vi "GetCmapArrays.vi"() -> (0 "Parula Array":u32[](array[numeric])=[4073128, 4073388, 4139183, 4139442, 4205236, 4205495, 4271290, 4271549, 4337343, 4337602, 4403397, 4403656, 4403914, 4469709, 4469968, 4535762, 4536277, 4536535, 4602329, 4602588, 4602846, 4603360, 4669153, 4669411, 4669925, 4670182, 4670696, 4670953, 4671211, 4737260, 4737517, 4738030, 4738288, 4738801, 4739058, 4739315, 4739828, 4740085, 4740342, 4675319, 4675575, 4676088, 4676345, 4676602, 4677114, 4611835, 4612347, 4612604, 4547324, 4547837, 4482557, 4417533, 4417790, 4352766, 4287486, 4222462, 4157183, 4092159, 3961343, 3896319, 3765503, 3700478, 3569662, 3504637, 3373821, 3308796, 3243516, 3178491, 3113210, 3113722, 3048441, 3048696, 3049208, 3049463, 2984182, 2984693, 2984948, 2985203, 2985714, 2920433, 2920688, 2855407, 2790382, 2725101, 2659820, 2594795, 2595050, 2529769, 2530024, 2464744, 2464999, 2399974, 2400229, 2334949, 2335204, 2269924, 2204643, 2139619, 2074338, 2009057, 1943777, 1944032, 1878751, 1813470, 1748189, 1682908, 1552090, 1486809, 1355992, 1225174, 1094357, 963540, 766930, 570577, 439759, 308942, 178124, 112586, 47305, 47559, 47814, 113348, 179138, 310209, 441535, 638397, 900540, 1097402, 1359544, 1556406, 1753269, 1949875, 2146737, 2343343, 2474670, 2605740, 2737066, 2868136, 2933926, 3064997, 3130787, 3261857, 3327647, 3393437, 3524507, 3590297, 3721366, 3787156, 3918226, 4049552, 4246157, 4377227, 4574089, 4770694, 4967300, 5164161, 5360767, 5557372, 5753978, 5950583, 6212980, 6409586, 6606191, 6802796, 7064937, 7261542, 7523684, 7785569, 7982174, 8244315, 8506457, 8703062, 8964947, 9161553, 9423694, 9685579, 9882184, 10144070, 10340675, 10602560, 10799166, 10995515, 11257657, 11454007, 11716149, 11912499, 12108849, 12305455, 12501805, 12763948, 12960298, 13156649, 13353256, 13549607, 13680423, 13877031, 14073383, 14269992, 14400808, 14597161, 14793770, 14924843, 15121197, 15252270, 15383088, 15514162, 15710773, 15841847, 15972921, 16103995, 16235069, 16366142, 16497470, 16563262, 16694589, 16694844, 16695355, 16695610, 16695865, 16696376, 16696631, 16697141, 16697396, 16697907, 16632626, 16633137, 16633393, 16568368, 16503343, 16503598, 16438574, 16373293, 16373804, 16308523, 16243498, 16244010, 16178729, 16179240, 16113960, 16114471, 16114982, 16115238, 16115749, 16116004, 16116515, 16116770, 16117281, 16183072, 16183583, 16183838, 16249884, 16250139, 16316186, 16316440, 16382230, 16382741], 1 "Viridis Array":u32[](array[numeric])=[4456788, 4457046, 4523095, 4523353, 4589402, 4589660, 4590173, 4590430, 4656480, 4656737, 4657251, 4657508, 4658021, 4723815, 4724328, 4724585, 4724842, 4725356, 4725613, 4725870, 4726127, 4726640, 4726897, 4727155, 4727668, 4727925, 4728182, 4728439, 4728952, 4729209, 4663930, 4664442, 4664699, 4664956, 4665213, 4599934, 4600446, 4600703, 4600960, 4535681, 4536193, 4536450, 4471171, 4471427, 4471684, 4406660, 4406917, 4341637, 4341894, 4342150, 4276871, 4277383, 4212104, 4212360, 4147080, 4147337, 4082057, 4082313, 4082826, 4017546, 4017802, 3952522, 3952779, 3887499, 3887755, 3822475, 3822732, 3757452, 3757708, 3692684, 3692940, 3627660, 3627917, 3562637, 3562893, 3497613, 3497869, 3432589, 3432845, 3367565, 3367821, 3302542, 3302798, 3237518, 3237774, 3238030, 3172750, 3173006, 3107726, 3107982, 3042702, 3042958, 3043214, 2977934, 2978190, 2912654, 2912910, 2913166, 2847886, 2848142, 2782862, 2783118, 2783374, 2718094, 2718350, 2718606, 2653326, 2653582, 2588302, 2588558, 2588814, 2523534, 2523790, 2523790, 2458510, 2458766, 2459022, 2393742, 2393998, 2328718, 2328974, 2329229, 2263949, 2264205, 2264461, 2199181, 2199437, 2199693, 2199948, 2134668, 2134668, 2134924, 2069644, 2069899, 2070155, 2070411, 2070667, 2070922, 2071178, 2005898, 2006153, 2006409, 2072201, 2072456, 2072712, 2072968, 2072967, 2073223, 2139014, 2139270, 2205061, 2205317, 2271109, 2271364, 2337155, 2402947, 2468738, 2468994, 2534785, 2600321, 2666112, 2731903, 2797695, 2929022, 2994813, 3060604, 3126396, 3257723, 3323514, 3454585, 3520377, 3651704, 3717495, 3848822, 3914613, 4045940, 4177011, 4242802, 4374129, 4505456, 4636783, 4768110, 4899181, 5030508, 5161835, 5293162, 5424489, 5555560, 5686887, 5818213, 5949540, 6080611, 6211938, 6343264, 6540127, 6671198, 6802524, 6933851, 7130458, 7261784, 7393111, 7589974, 7721044, 7852371, 8048977, 8180304, 8377166, 8508237, 8705099, 8836425, 9033032, 9164358, 9360965, 9492291, 9688897, 9820224, 10016830, 10213692, 10344763, 10541625, 10672695, 10869558, 11066164, 11197490, 11394096, 11590959, 11722029, 11918891, 12115497, 12246568, 12443430, 12640037, 12771107, 12967969, 13164576, 13295903, 13492509, 13689116, 13820443, 14017050, 14213657, 14344985, 14541592, 14672664, 14869528, 15066137, 15197209, 15394074, 15525147, 15721756, 15852829, 16049694, 16180768, 16311841, 16508707, 16639781], 2 "Hot Array":u32[](array[numeric])=[196608, 327680, 524288, 720896, 851968, 1048576, 1245184, 1376256, 1572864, 1769472, 1900544, 2097152, 2293760, 2424832, 2621440, 2752512, 2949120, 3145728, 3276800, 3473408, 3670016, 3801088, 3997696, 4194304, 4325376, 4521984, 4718592, 4849664, 5046272, 5242880, 5373952, 5570560, 5767168, 5898240, 6094848, 6291456, 6422528, 6619136, 6815744, 6946816, 7143424, 7340032, 7471104, 7667712, 7864320, 7995392, 8192000, 8388608, 8519680, 8716288, 8847360, 9043968, 9240576, 9371648, 9568256, 9764864, 9895936, 10092544, 10289152, 10420224, 10616832, 10813440, 10944512, 11141120, 11337728, 11468800, 11665408, 11862016, 11993088, 12189696, 12386304, 12517376, 12713984, 12910592, 13041664, 13238272, 13434880, 13565952, 13762560, 13893632, 14090240, 14286848, 14417920, 14614528, 14811136, 14942208, 15138816, 15335424, 15466496, 15663104, 15859712, 15990784, 16187392, 16384000, 16515072, 16711680, 16712448, 16712960, 16713728, 16714496, 16715008, 16715776, 16716544, 16717056, 16717824, 16718592, 16719104, 16719872, 16720640, 16721152, 16721920, 16722432, 16723200, 16723968, 16724480, 16725248, 16726016, 16726528, 16727296, 16728064, 16728576, 16729344, 16730112, 16730624, 16731392, 16732160, 16732672, 16733440, 16734208, 16734720, 16735488, 16736256, 16736768, 16737536, 16738304, 16738816, 16739584, 16740352, 16740864, 16741632, 16742400, 16742912, 16743680, 16744448, 16744960, 16745728, 16746240, 16747008, 16747776, 16748288, 16749056, 16749824, 16750336, 16751104, 16751872, 16752384, 16753152, 16753920, 16754432, 16755200, 16755968, 16756480, 16757248, 16758016, 16758528, 16759296, 16760064, 16760576, 16761344, 16762112, 16762624, 16763392, 16764160, 16764672, 16765440, 16765952, 16766720, 16767488, 16768000, 16768768, 16769536, 16770048, 16770816, 16771584, 16772096, 16772864, 16773632, 16774144, 16774912, 16775680, 16776192, 16776960, 16776964, 16776968, 16776972, 16776976, 16776980, 16776984, 16776988, 16776992, 16776996, 16777000, 16777004, 16777008, 16777012, 16777016, 16777020, 16777024, 16777028, 16777032, 16777036, 16777040, 16777044, 16777048, 16777052, 16777056, 16777060, 16777064, 16777068, 16777072, 16777076, 16777080, 16777084, 16777088, 16777091, 16777095, 16777099, 16777103, 16777107, 16777111, 16777115, 16777119, 16777123, 16777127, 16777131, 16777135, 16777139, 16777143, 16777147, 16777151, 16777155, 16777159, 16777163, 16777167, 16777171, 16777175, 16777179, 16777183, 16777187, 16777191, 16777195, 16777199, 16777203, 16777207, 16777211, 16777215], 3 "Plasma Array":u32[](array[numeric])=[854151, 1050504, 1247113, 1443722, 1640076, 1771149, 1902222, 2098831, 2229904, 2360977, 2491793, 2622866, 2753939, 2885012, 3016085, 3081622, 3212695, 3343767, 3474584, 3605657, 3671194, 3802266, 3933339, 4064412, 4129948, 4261021, 4391838, 4457374, 4588447, 4719519, 4785056, 4916129, 4981409, 5112482, 5243554, 5309091, 5440163, 5571236, 5636516, 5767588, 5833125, 5964197, 6029734, 6160806, 6291878, 6357159, 6488231, 6553767, 6684839, 6750376, 6881448, 6946984, 7078056, 7209128, 7274664, 7405736, 7471528, 7602600, 7668136, 7799208, 7864744, 7996072, 8061608, 8192936, 8258472, 8389800, 8455335, 8586663, 8652199, 8783526, 8849318, 8915110, 9046437, 9112229, 9243557, 9309348, 9375140, 9506467, 9572259, 9703586, 9769377, 9835425, 9966752, 10032543, 10098335, 10229662, 10295453, 10361245, 10492572, 10558363, 10624410, 10690202, 10821529, 10887320, 10953111, 11018902, 11150229, 11216020, 11282068, 11347859, 11413650, 11544977, 11610768, 11676559, 11742350, 11808397, 11874188, 11939979, 12005770, 12071561, 12202888, 12268680, 12334471, 12400518, 12466309, 12532100, 12597891, 12663682, 12729473, 12795264, 12861055, 12927102, 12992893, 13058684, 13124475, 13190266, 13256058, 13321849, 13387640, 13388151, 13453942, 13519733, 13585524, 13651315, 13717106, 13782897, 13848945, 13914736, 13980527, 13980782, 14046573, 14112364, 14178155, 14243946, 14309994, 14310249, 14376040, 14441831, 14507622, 14573413, 14573924, 14639715, 14705507, 14771298, 14837089, 14837344, 14903391, 14969182, 15034973, 15035229, 15101020, 15167067, 15167322, 15233113, 15298904, 15299159, 15365207, 15430998, 15431253, 15497044, 15563091, 15563346, 15629137, 15694929, 15695440, 15761231, 15761486, 15827277, 15827788, 15893579, 15959371, 15959882, 16025673, 16025928, 16091975, 16092230, 16158021, 16158532, 16224324, 16224579, 16225090, 16290881, 16291136, 16357183, 16357438, 16357950, 16423741, 16423996, 16424507, 16490298, 16490809, 16491064, 16556856, 16557367, 16557622, 16558133, 16558388, 16624435, 16624691, 16625202, 16625457, 16625968, 16626223, 16626735, 16626990, 16693037, 16693292, 16693804, 16694059, 16694570, 16694826, 16695337, 16630313, 16630568, 16631079, 16631335, 16631847, 16632358, 16632614, 16567589, 16567845, 16568357, 16568869, 16503588, 16504100, 16504612, 16439332, 16439844, 16374820, 16375077, 16310053, 16310565, 16245285, 16245797, 16180774, 16181286, 16116006, 16116519, 16051495, 15986215, 15986727, 15921703, 15856678, 15856933, 15791908, 15792417], 4 "Jet Array":u32[](array[numeric])=[131, 135, 139, 143, 147, 151, 155, 159, 163, 167, 171, 175, 179, 183, 187, 191, 195, 199, 203, 207, 211, 215, 219, 223, 227, 231, 235, 239, 243, 247, 251, 255, 1279, 2303, 3327, 4351, 5375, 6399, 7423, 8447, 9471, 10495, 11519, 12543, 13567, 14591, 15615, 16639, 17663, 18687, 19711, 20735, 21759, 22783, 23807, 24831, 25855, 26879, 27903, 28927, 29951, 30975, 31999, 33023, 33791, 34815, 35839, 36863, 37887, 38911, 39935, 40959, 41983, 43007, 44031, 45055, 46079, 47103, 48127, 49151, 50175, 51199, 52223, 53247, 54271, 55295, 56319, 57343, 58367, 59391, 60415, 61439, 62463, 63487, 64511, 65535, 327675, 589815, 851955, 1114095, 1376235, 1638375, 1900515, 2162655, 2424795, 2686935, 2949075, 3211215, 3473355, 3735495, 3997635, 4259775, 4521915, 4784055, 5046195, 5308335, 5570475, 5832615, 6094755, 6356895, 6619035, 6881175, 7143315, 7405455, 7667595, 7929735, 8191875, 8454016, 8650620, 8912760, 9174900, 9437040, 9699180, 9961320, 10223460, 10485600, 10747740, 11009880, 11272020, 11534160, 11796300, 12058440, 12320580, 12582720, 12844860, 13107000, 13369140, 13631280, 13893420, 14155560, 14417700, 14679840, 14941980, 15204120, 15466260, 15728400, 15990540, 16252680, 16514820, 16776960, 16775936, 16774912, 16773888, 16772864, 16771840, 16770816, 16769792, 16768768, 16767744, 16766720, 16765696, 16764672, 16763648, 16762624, 16761600, 16760576, 16759552, 16758528, 16757504, 16756480, 16755456, 16754432, 16753408, 16752384, 16751360, 16750336, 16749312, 16748288, 16747264, 16746240, 16745216, 16744448, 16743424, 16742400, 16741376, 16740352, 16739328, 16738304, 16737280, 16736256, 16735232, 16734208, 16733184, 16732160, 16731136, 16730112, 16729088, 16728064, 16727040, 16726016, 16724992, 16723968, 16722944, 16721920, 16720896, 16719872, 16718848, 16717824, 16716800, 16715776, 16714752, 16713728, 16712704, 16711680, 16449536, 16187392, 15925248, 15663104, 15400960, 15138816, 14876672, 14614528, 14352384, 14090240, 13828096, 13565952, 13303808, 13041664, 12779520, 12517376, 12255232, 11993088, 11730944, 11468800, 11206656, 10944512, 10682368, 10420224, 10158080, 9895936, 9633792, 9371648, 9109504, 8847360, 8585216, 8388608], 5 "Grayscale Array":u32[](array[numeric])=[0, 65793, 131586, 197379, 263172, 328965, 394758, 460551, 526344, 592137, 657930, 723723, 789516, 855309, 921102, 986895, 1052688, 1118481, 1184274, 1250067, 1315860, 1381653, 1447446, 1513239, 1579032, 1644825, 1710618, 1776411, 1842204, 1907997, 1973790, 2039583, 2105376, 2171169, 2236962, 2302755, 2368548, 2434341, 2500134, 2565927, 2631720, 2697513, 2763306, 2829099, 2894892, 2960685, 3026478, 3092271, 3158064, 3223857, 3289650, 3355443, 3421236, 3487029, 3552822, 3618615, 3684408, 3750201, 3815994, 3881787, 3947580, 4013373, 4079166, 4144959, 4210752, 4276545, 4342338, 4408131, 4473924, 4539717, 4605510, 4671303, 4737096, 4802889, 4868682, 4934475, 5000268, 5066061, 5131854, 5197647, 5263440, 5329233, 5395026, 5460819, 5526612, 5592405, 5658198, 5723991, 5789784, 5855577, 5921370, 5987163, 6052956, 6118749, 6184542, 6250335, 6316128, 6381921, 6447714, 6513507, 6579300, 6645093, 6710886, 6776679, 6842472, 6908265, 6974058, 7039851, 7105644, 7171437, 7237230, 7303023, 7368816, 7434609, 7500402, 7566195, 7631988, 7697781, 7763574, 7829367, 7895160, 7960953, 8026746, 8092539, 8158332, 8224125, 8289918, 8355711, 8421504, 8487297, 8553090, 8618883, 8684676, 8750469, 8816262, 8882055, 8947848, 9013641, 9079434, 9145227, 9211020, 9276813, 9342606, 9408399, 9474192, 9539985, 9605778, 9671571, 9737364, 9803157, 9868950, 9934743, 10000536, 10066329, 10132122, 10197915, 10263708, 10329501, 10395294, 10461087, 10526880, 10592673, 10658466, 10724259, 10790052, 10855845, 10921638, 10987431, 11053224, 11119017, 11184810, 11250603, 11316396, 11382189, 11447982, 11513775, 11579568, 11645361, 11711154, 11776947, 11842740, 11908533, 11974326, 12040119, 12105912, 12171705, 12237498, 12303291, 12369084, 12434877, 12500670, 12566463, 12632256, 12698049, 12763842, 12829635, 12895428, 12961221, 13027014, 13092807, 13158600, 13224393, 13290186, 13355979, 13421772, 13487565, 13553358, 13619151, 13684944, 13750737, 13816530, 13882323, 13948116, 14013909, 14079702, 14145495, 14211288, 14277081, 14342874, 14408667, 14474460, 14540253, 14606046, 14671839, 14737632, 14803425, 14869218, 14935011, 15000804, 15066597, 15132390, 15198183, 15263976, 15329769, 15395562, 15461355, 15527148, 15592941, 15658734, 15724527, 15790320, 15856113, 15921906, 15987699, 16053492, 16119285, 16185078, 16250871, 16316664, 16382457, 16448250, 16514043, 16579836, 16645629, 16711422, 16777215])   [LabVIEW 2015]
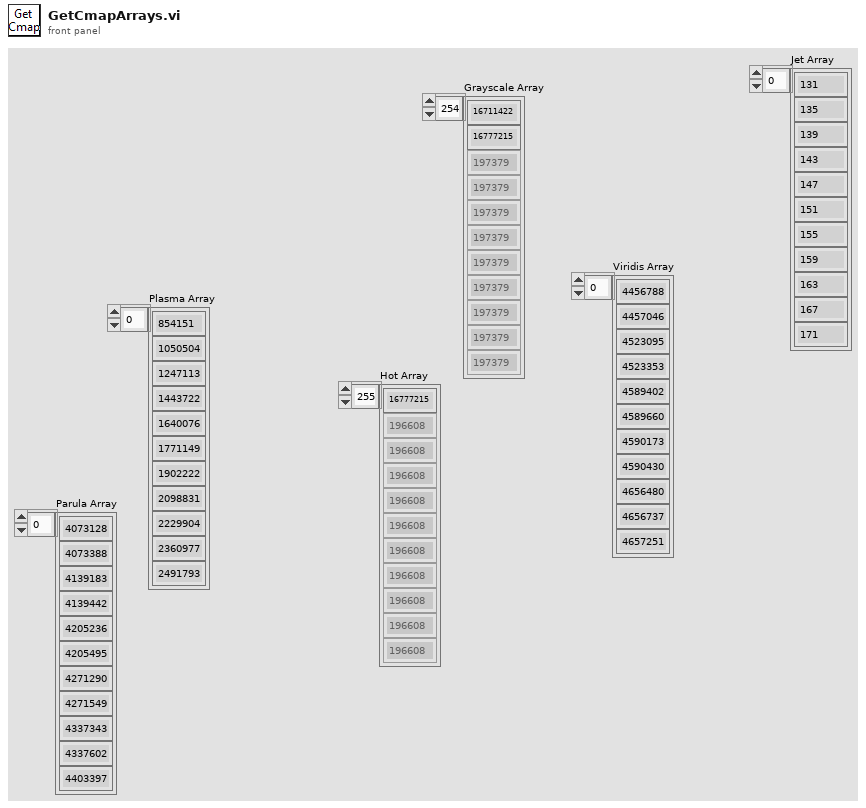
[diagram p1: front panel]
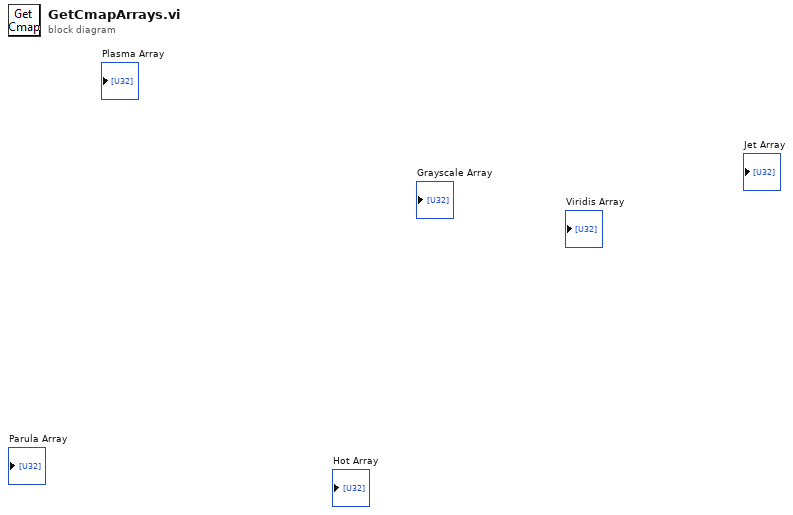
[diagram p0: block diagram]
diagram:
